vi "Parse Structure Names.vi"(8 "Error In":errorcluster, 9 "Data":string, 10 "Structure IDs":string[](array[string]), 11 "Nest Config":T1) -> (0 "Error Out":errorcluster, 1 "Data":string, 2 "Structure Names":string[](array[string]), 3 "Nest Config":T1)   [LabVIEW 2013, in "LMH-Nest.lvlib"]
uses:
  LMH-Nest.lvlib
  Type Defs/Nest Config.ctl
  <vilib>/httpClient/ClientHandle.ctl
  Type Defs/Session Data.ctl
  <vilib>/httpClient/LabVIEWHTTPClient.lvlib
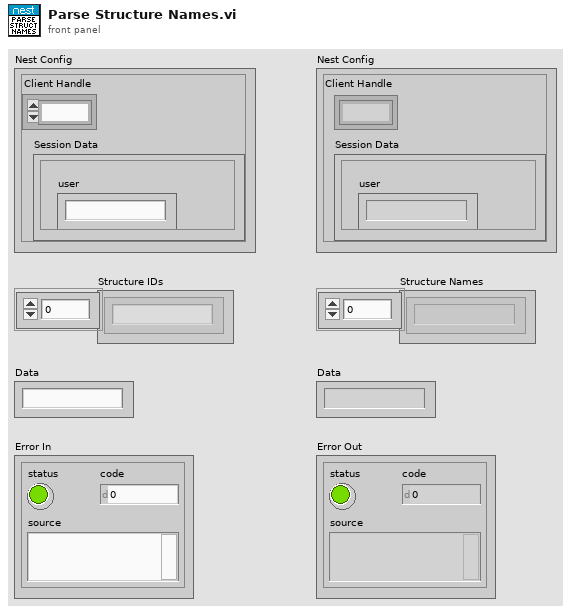
[diagram p1: front panel]
types:
  T1 = typedef "LMH-Nest.lvlib/Nest Config.ctl" = cluster{"Client Handle":T2, "Session Data":T3}
  T2 = typedef "LabVIEWHTTPClient.lvlib/ClientHandle.ctl" = refnum<k1>
  T3 = typedef "LMH-Nest.lvlib/Session Data.ctl" = cluster{"is_superuser":bool, "is_staff":bool, "urls":cluster{"transport_url":string, "rubyapi_url":string, "weather_url":string, "log_upload_url":string, "support_url":string}, "limits":cluster{"thermostats_per_structure":u32, "structures":u32, "thermostats":u32, "smoke_detectors":u32, "smoke_detectors_per_structure":u32}, "access_token":string, "userid":string, "expires_in":string, "email":string, "user":string, "language":string}
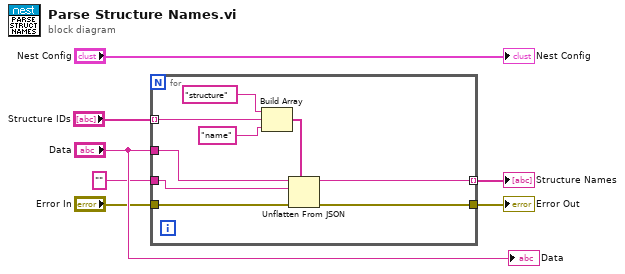
[diagram p0: block diagram]
diagram:
  n1 = for {
    tunnel: [w16] -> w6
    tunnel: "Data" -> [w15]
    tunnel: "Error In" -> [w12]
    tunnel: "" -> [w11]
    tunnel: "Structure IDs" -> [w10] mode=indexing
    tunnel: [w9] -> w1 mode=indexing
    n2 = Build Array("structure", w10, "name" ("element")) -> (w14:string[])
    n3 = Unflatten From JSON(path=w14, JSON string=w15, type and defaults=w11, error in (no error)=w12) -> (value=w9:string, error out=w16:errorcluster)  [unwired: 3 in]
  }
  "Error Out" <- w6
  "Structure Names" <- w1
  "Data" <- "Data"
  "Nest Config" <- "Nest Config"
